vi "ReadNamesNode.vi"(8 "Error In":errorcluster, 11 "Keithley2602 Node In":refnum<k20>) -> (0 "Error Out":errorcluster, 2 "Names":string[][](array[string]), 3 "Keithley2602 Node Out":refnum<k20>)   [LabVIEW 2013]
uses:
  <vilib>/xml/NI_XML.lvlib
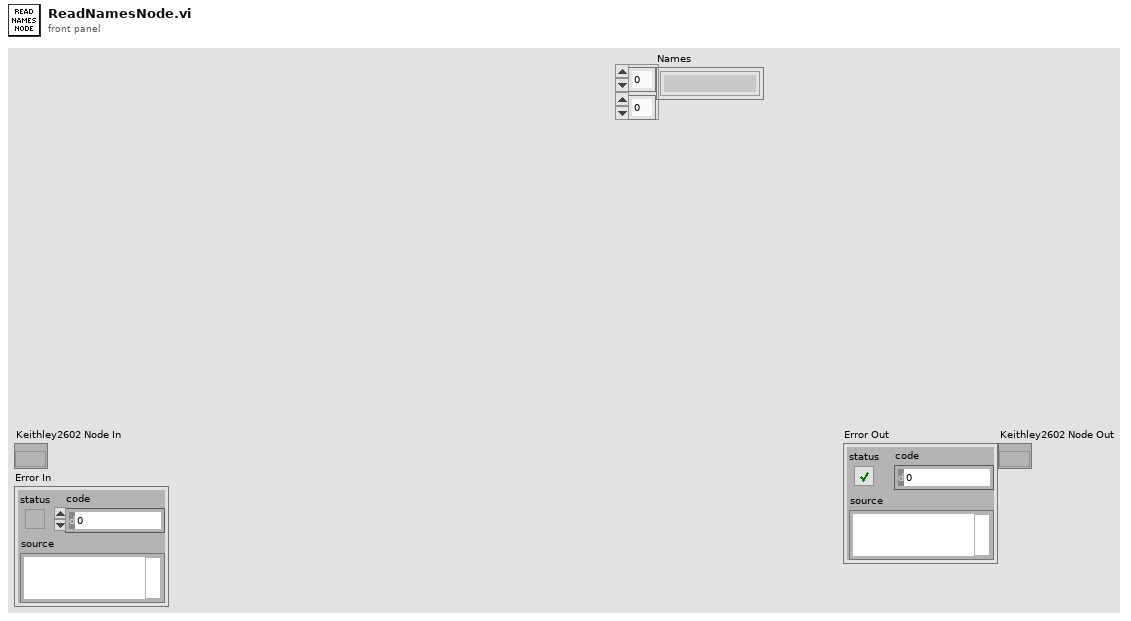
[diagram p1: front panel]
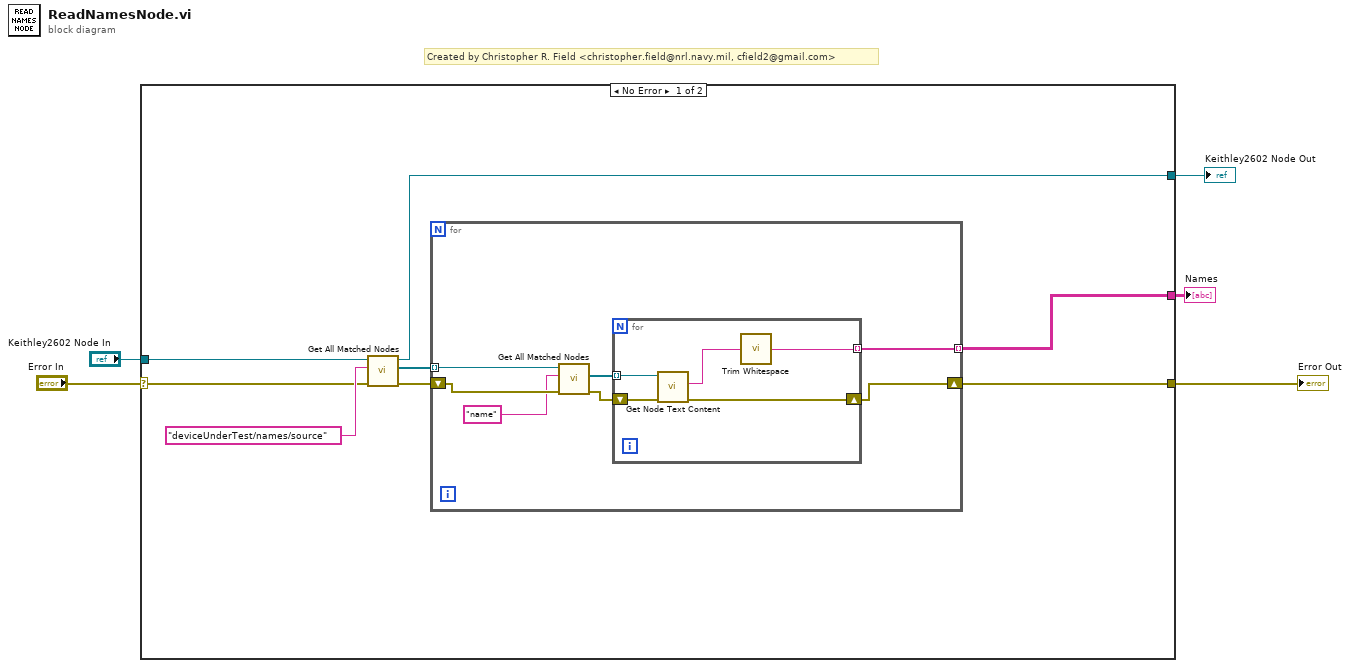
[diagram p0: block diagram]
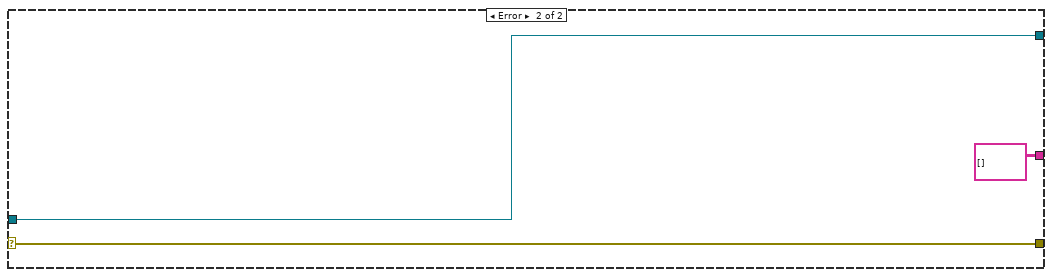
[diagram p2: hidden frame]
diagram:
  # "Created by Christopher R. Field <christopher.field@nrl.navy.mil, cfield2@gmail.com>"
  n1 = case shown="No Error" "Error In" {
    selector: "Error In" -> [w7 w27]
    tunnel: "Keithley2602 Node In" -> [w10 w28]
    tunnel: [w9 w27] -> w4
    tunnel: [w8 w28] -> w3
    tunnel: [w6 string[][] []] -> w1
    frame No Error {
      n2 = call <vilib>:"Get All Matched Nodes.vi"("error in (no error)"=w7, "XPath expression"="deviceUnderTest/names/source", "node in"=w10) -> ("error out"=w11:errorcluster, "node result array"=w12:refnum<k20>[], "node out"=w8:refnum<k20>)  [unwired: 6 in]
      n3 = for {
        tunnel: w12 -> [w20] mode=indexing
        shift-right: [w15] -> w9
        shift-left: w11 -> [w19]
        tunnel: [w14] -> w6 mode=indexing
        n4 = call <vilib>:"Get All Matched Nodes.vi"("error in (no error)"=w19, "XPath expression"="name", "node in"=w20) -> ("error out"=w16:errorcluster, "node result array"=w17:refnum<k20>[])  [unwired: 6 in, 1 out]
        n5 = for {
          tunnel: w17 -> [w24] mode=indexing
          shift-right: [w25] -> w15
          shift-left: w16 -> [w23]
          tunnel: [w21] -> w14 mode=indexing
          n6 = call <vilib>:"Get Node Text Content.vi"("error in (no error)"=w23, "node in"=w24) -> ("error out"=w25:errorcluster, "node text"=w22:string)  [unwired: 7 in, 1 out]
          n7 = call <vilib>:"Trim Whitespace.vi"("string"=w22) -> ("trimmed string"=w21:string)  [unwired: 1 in]
        }
      }
    }
    frame Error {
    }
  }
  "Error Out" <- w4
  "Keithley2602 Node Out" <- w3
  "Names" <- w1
